vi "Lab14_PC.vi"() -> ()   [LabVIEW 2016]
uses:
  <vilib>/National Instruments/IoT Education Toolkit Beta/TW API/TW_Gadgets_Boolean.vi
  <vilib>/National Instruments/IoT Education Toolkit Beta/TW API/TW_Gadgets_Text.vi
  <vilib>/National Instruments/IoT Education Toolkit Beta/TW API/TW_Gadget_Number.vi
  <vilib>/National Instruments/IoT Education Toolkit Beta/TW API/TW_SetPropertyValue_String_Edit.vi
  <vilib>/National Instruments/IoT Education Toolkit Beta/TW API/TW_SetPropertyValue_Int_Edit.vi
  <vilib>/National Instruments/IoT Education Toolkit Beta/TW API/Properties.lvclass
  <vilib>/National Instruments/IoT Education Toolkit Beta/TW API/Thing.lvclass
  <vilib>/National Instruments/IoT Education Toolkit Beta/TW API/Gadget.lvclass
panel:
  out "CounterBennett":i64
  out "URL":string[](array[string])
  in  "Stop":bool
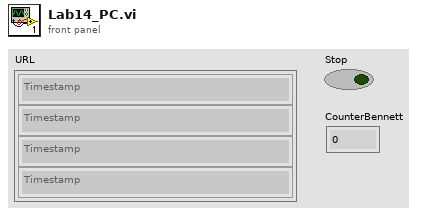
[diagram p1: front panel]
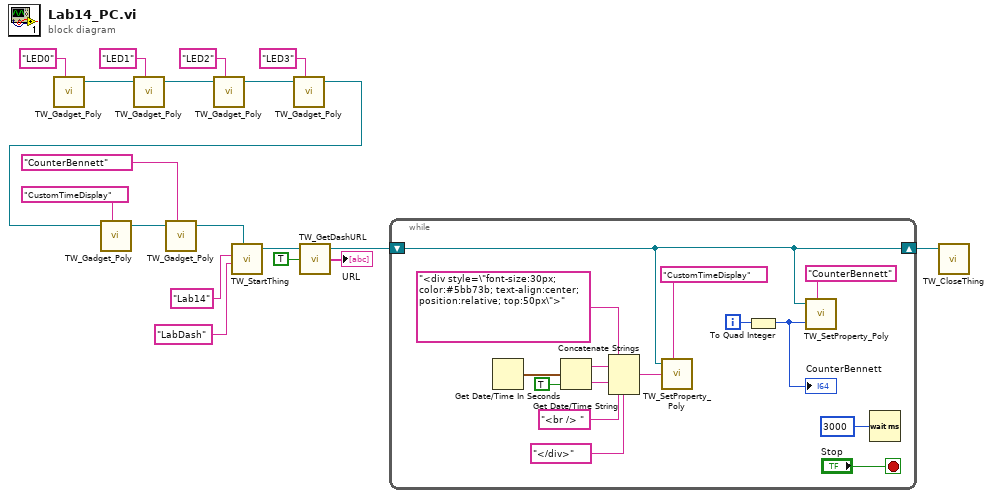
[diagram p0: block diagram]
diagram:
  n1 = call-poly <vilib>:"TW_Gadget_Poly.vi"("Property to display"="LED0") -> ("Gadgets out"=w6:refnum<class "Gadget.lvclass">)  [unwired: 6 in]
  n2 = call-poly <vilib>:"TW_Gadget_Poly.vi"("Gadgets in"=w6, "Property to display"="LED1") -> ("Gadgets out"=w2:refnum<class "Gadget.lvclass">)  [unwired: 5 in]
  n3 = call-poly <vilib>:"TW_Gadget_Poly.vi"("Gadgets in"=w2, "Property to display"="LED2") -> ("Gadgets out"=w3:refnum<class "Gadget.lvclass">)  [unwired: 5 in]
  n4 = call-poly <vilib>:"TW_Gadget_Poly.vi"("Gadgets in"=w3, "Property to display"="LED3") -> ("Gadgets out"=w1:refnum<class "Gadget.lvclass">)  [unwired: 5 in]
  n5 = call-poly <vilib>:"TW_Gadget_Poly.vi"("Gadgets in"=w1, "Property to display"="CustomTimeDisplay") -> ("Gadgets out"=w13:refnum<class "Gadget.lvclass">)  [unwired: 5 in]
  n6 = call-poly <vilib>:"TW_Gadget_Poly.vi"("Gadgets in"=w13, "Property to display"="CounterBennett") -> ("Gadgets out"=w11:refnum<class "Gadget.lvclass">)  [unwired: 5 in]
  n7 = call <vilib>:"TW_StartThing.vi"("Gadgets"=w11, "ThingName"="Lab14", "Dashboard"="LabDash") -> ("Thing Out"=w17:refnum<class "Thing.lvclass">)  [unwired: 3 in, 2 out]
  n8 = call <vilib>:"TW_GetDashURL.vi"("Thing In"=w17, "Open Webpage?"=TRUE) -> ("Thing Out"=w16:refnum<class "Thing.lvclass">, "Links"=→"URL":string[])  [unwired: 3 in, 1 out]
  n9 = while {
    shift-right: [w20] -> w12
    shift-left: w16 -> [w20]
    i -> [w27]
    stop <- "Stop" stop-if-true
    n10 = Get Date/Time In Seconds() -> (seconds since 1Jan1904=w31:timestamp)
    n11 = Get Date/Time String(seconds (now)=w31, want seconds? (F)=TRUE) -> (date string=w30:string, time string=w29:string)  [unwired: 1 in]
    n12 = Concatenate Strings("<div style=\"font-size:30px; color:#5bb73b; text-align:center; position:relative; top:50px\">", w30, "<br /> ", w29, "</div>") -> (w24:string)
    n13 = call-poly <vilib>:"TW_SetProperty_Poly.vi"("Thing in"=w20, "Property name"="CustomTimeDisplay", "Value"=w24) -> ()  [unwired: 3 in, 2 out]
    n14 = To Quad Integer(1:w27) -> (0:w25:i64)
    "CounterBennett" <- w25
    n15 = call-poly <vilib>:"TW_SetProperty_Poly.vi"("Thing in"=w20, "Property name"="CounterBennett", "Value"=w25) -> ()  [unwired: 3 in, 2 out]
    n16 = Wait (ms)(milliseconds to wait=u32 3000) -> ()  [unwired: 1 out]
  }
  n17 = call <vilib>:"TW_CloseThing.vi"("Thing In"=w12) -> ()  [unwired: 6 in, 1 out]
